vi "Finalize.vi"(8 "error in (no error)":errorcluster, 11 "User Interface in":refnum<class "User Interface.lvclass">) -> (0 "error out":errorcluster, 1 "data version":T1, 2 "data":string, 3 "User Interface out":refnum<class "User Interface.lvclass">)   [LabVIEW 2017, in "DSF Core.lvlib" / "User Interface.lvclass"]
uses:
  User Interface.lvclass
  Configuration/Configuration.lvclass
  Typedefs/DSF Version Info.ctl
  DSF Core.lvlib
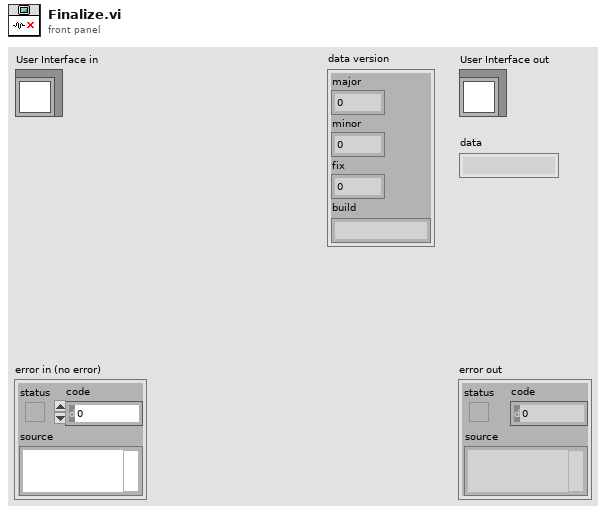
[diagram p1: front panel]
types:
  T1 = typedef "DSF Core.lvlib/DSF Version Info.ctl" = cluster{"major":u32, "minor":u32, "fix":u32, "build":string}
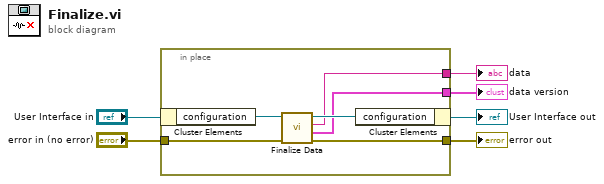
[diagram p0: block diagram]
diagram:
  n1 = in-place {
    in-place-border: "error in (no error)" -> [w10]
    in-place-border: [w9] -> w4
    in-place-border: [w7] -> w2
    in-place-border: [w8] -> w1
    n2 = in-place-cluster #1("User Interface in") -> ("configuration"=w12:refnum<class "Configuration.lvclass">)
    n3 = call-dynamic "Finalize Data.vi"("error in (no error)"=w10, "Configuration in"=w12) -> ("error out"=w9:errorcluster, "data version"=w7:T1, "data"=w8:string, "Configuration out"=w11:refnum<class "Configuration.lvclass">)  [unwired: 6 in]
    n4 = in-place-cluster #1("configuration"=w11) -> (→"User Interface out":refnum<class "User Interface.lvclass">)
  }
  "error out" <- w4
  "data version" <- w2
  "data" <- w1
